vi "RTS Polarity CMD.vi"(7 "Station":u16=1 min=1 max=8 step=1, 8 "Error In":errorcluster, 11 "NewVal":T1) -> (0 "Error Out":errorcluster, 3 "Polarity CMD":string)   [LabVIEW 2016]
uses:
  Drivers/WAGO 750-881/Type Definitions/Wago Polarity Selector.ctl
  Drivers/WAGO 750-881/Type Definitions/Wago Input Commands.ctl
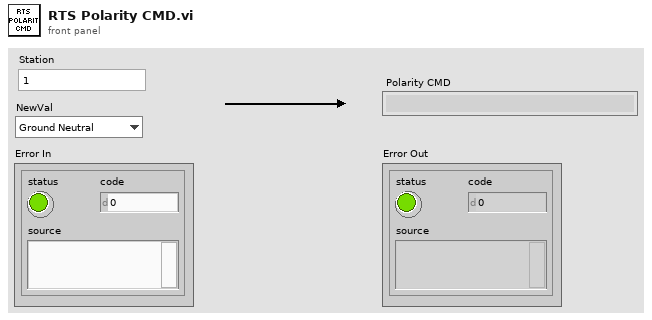
[diagram p1: front panel]
types:
  T1 = typedef "Wago Polarity Selector.ctl" = enum16{"Ground Neutral", "Ground Line"}
  T2 = typedef "Wago Input Commands.ctl" = u16
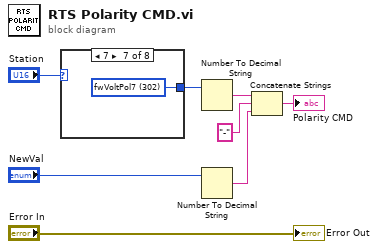
[diagram p0: block diagram]
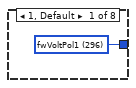
[diagram p2: hidden frame]
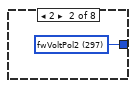
[diagram p3: hidden frame]
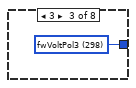
[diagram p4: hidden frame]
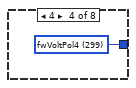
[diagram p5: hidden frame]
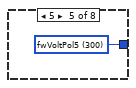
[diagram p6: hidden frame]
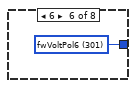
[diagram p7: hidden frame]
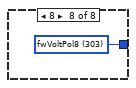
[diagram p8: hidden frame]
diagram:
  n1 = case shown="7" "Station" {
    tunnel: [w9 w10 w11 w12 w13 w14 w15 w16] -> w6
    frame 1, Default {
      w9 = T2 296 items=["fwS1Volt1"=0, "fwS1Volt2"=1, "fwS2Volt1"=2, "fwS2Volt2"=3, "fwS3Volt1"=4, "fwS3Volt2"=5, "fwS4Volt1"=6, "fwS4Volt2"=7, "fwS5Volt1"=8, "fwS5Volt2"=9, "fwS6Volt1"=10, "fwS6Volt2 "=11, "fwS7Volt1"=12, "fwS7Volt2"=13, "fwS8Volt1"=14, "fwS8Volt2"=15, "fwRoomHum"=16, "fwRoomTemp"=17, "fwAISpare1"=18, "fwAISpare2"=19, "fwSuppTemp"=20, "fwCoolTemp"=21, "fwDehumTemp"=22, "fwUnused"=23, "Bool Inputs"=24, "gwVoltRate1"=256, "gwVoltRate2"=257, "gwVoltRate3"=258, "gwVoltRate4"=259, "gwVoltRate5"=260, "gwVoltRate6"=261, "gwVoltRate7"=262, "gwVoltRate8"=263, "gwVoltWindow5/1"=264, "gwVoltWindow6/2"=265, "gwVoltWindow7/3"=266, "gwVoltWindow8/4"=267, "fwVoltSet1"=272, "fwVoltSet2"=273, "fwVoltSet3"=274, "fwVoltSet4"=275, "fwVoltSet5"=276, "fwVoltSet6"=277, "fwVoltSet7"=278, "fwVoltSet8"=279, "fwVoltRng1"=280, "fwVoltRng2"=281, "fwVoltRng3"=282, "fwVoltRng4"=283, "fwVoltRng5"=284, "fwVoltRng6"=285, "fwVoltRng7"=286, "fwVoltRng8"=287, "fwVoltPol1"=296, "fwVoltPol2"=297, "fwVoltPol3"=298, "fwVoltPol4"=299, "fwVoltPol5"=300, "fwVoltPol6"=301, "fwVoltPol7"=302, "fwVoltPol8"=303, "Rm1St1Dr1Cmd"=304, "Rm1St2Dr1Cmd"=305, "Rm1St3Dr1Cmd"=306, "Rm1St4Dr1Cmd"=307, "Rm1St5Dr1Cmd"=308, "Rm1St6Dr1Cmd"=309, "Rm1St7Dr1Cmd"=310, "Rm1St8Dr1Cmd"=311, "Rm1St1Dr2Cmd"=312, "Rm1St2Dr2Cmd"=313, "Rm1St3Dr2Cmd"=314, "Rm1St4Dr2Cmd"=315, "Rm1St5Dr2Cmd"=316, "Rm1St6Dr2Cmd"=317, "Rm1St7Dr2Cmd"=318, "Rm1St8Dr2Cmd"=319, "Rm1St1Dr3Cmd"=320, "Rm1St2Dr3Cmd"=321, "Rm1St3Dr3Cmd"=322, "Rm1St4Dr3Cmd"=323, "Rm1St5Dr3Cmd"=324, "Rm1St6Dr3Cmd"=325, "Rm1St7Dr3Cmd"=326, "Rm1St8Dr3Cmd"=327, "fwRmTempSP"=328, "fwRmHumSP"=329, "fwCoolTempSP"=330, "fwDehumTempSP"=331, "fwRmRun"=332, "fwRmOk"=333, "fwTesting"=334, "fwRmDryP"=335, "fwRmDryI"=336, "fwRmHumP"=337, "fwRmHumI"=338, "fwRmHeatP"=339, "fwRmHeatI"=340, "fwCoolTempP"=341, "fwCoolTempI"=342, "fwDehumTempP"=343, "fwDehumTempI"=344, "fwGndLeak1"=345, "fwGndLeak2"=346, "fwGndLeak3"=347, "fwGndLeak4"=348, "fwGndLeak5"=349, "fwGndLeak6"=350, "fwGndLeak7"=351, "fwGndLeak8"=352, "Rm1OpenerCmd"=353] ("Ring")
    }
    frame 2 {
      w10 = T2 297 items=["fwS1Volt1"=0, "fwS1Volt2"=1, "fwS2Volt1"=2, "fwS2Volt2"=3, "fwS3Volt1"=4, "fwS3Volt2"=5, "fwS4Volt1"=6, "fwS4Volt2"=7, "fwS5Volt1"=8, "fwS5Volt2"=9, "fwS6Volt1"=10, "fwS6Volt2 "=11, "fwS7Volt1"=12, "fwS7Volt2"=13, "fwS8Volt1"=14, "fwS8Volt2"=15, "fwRoomHum"=16, "fwRoomTemp"=17, "fwAISpare1"=18, "fwAISpare2"=19, "fwSuppTemp"=20, "fwCoolTemp"=21, "fwDehumTemp"=22, "fwUnused"=23, "Bool Inputs"=24, "gwVoltRate1"=256, "gwVoltRate2"=257, "gwVoltRate3"=258, "gwVoltRate4"=259, "gwVoltRate5"=260, "gwVoltRate6"=261, "gwVoltRate7"=262, "gwVoltRate8"=263, "gwVoltWindow5/1"=264, "gwVoltWindow6/2"=265, "gwVoltWindow7/3"=266, "gwVoltWindow8/4"=267, "fwVoltSet1"=272, "fwVoltSet2"=273, "fwVoltSet3"=274, "fwVoltSet4"=275, "fwVoltSet5"=276, "fwVoltSet6"=277, "fwVoltSet7"=278, "fwVoltSet8"=279, "fwVoltRng1"=280, "fwVoltRng2"=281, "fwVoltRng3"=282, "fwVoltRng4"=283, "fwVoltRng5"=284, "fwVoltRng6"=285, "fwVoltRng7"=286, "fwVoltRng8"=287, "fwVoltPol1"=296, "fwVoltPol2"=297, "fwVoltPol3"=298, "fwVoltPol4"=299, "fwVoltPol5"=300, "fwVoltPol6"=301, "fwVoltPol7"=302, "fwVoltPol8"=303, "Rm1St1Dr1Cmd"=304, "Rm1St2Dr1Cmd"=305, "Rm1St3Dr1Cmd"=306, "Rm1St4Dr1Cmd"=307, "Rm1St5Dr1Cmd"=308, "Rm1St6Dr1Cmd"=309, "Rm1St7Dr1Cmd"=310, "Rm1St8Dr1Cmd"=311, "Rm1St1Dr2Cmd"=312, "Rm1St2Dr2Cmd"=313, "Rm1St3Dr2Cmd"=314, "Rm1St4Dr2Cmd"=315, "Rm1St5Dr2Cmd"=316, "Rm1St6Dr2Cmd"=317, "Rm1St7Dr2Cmd"=318, "Rm1St8Dr2Cmd"=319, "Rm1St1Dr3Cmd"=320, "Rm1St2Dr3Cmd"=321, "Rm1St3Dr3Cmd"=322, "Rm1St4Dr3Cmd"=323, "Rm1St5Dr3Cmd"=324, "Rm1St6Dr3Cmd"=325, "Rm1St7Dr3Cmd"=326, "Rm1St8Dr3Cmd"=327, "fwRmTempSP"=328, "fwRmHumSP"=329, "fwCoolTempSP"=330, "fwDehumTempSP"=331, "fwRmRun"=332, "fwRmOk"=333, "fwTesting"=334, "fwRmDryP"=335, "fwRmDryI"=336, "fwRmHumP"=337, "fwRmHumI"=338, "fwRmHeatP"=339, "fwRmHeatI"=340, "fwCoolTempP"=341, "fwCoolTempI"=342, "fwDehumTempP"=343, "fwDehumTempI"=344, "fwGndLeak1"=345, "fwGndLeak2"=346, "fwGndLeak3"=347, "fwGndLeak4"=348, "fwGndLeak5"=349, "fwGndLeak6"=350, "fwGndLeak7"=351, "fwGndLeak8"=352, "Rm1OpenerCmd"=353] ("Ring")
    }
    frame 3 {
      w11 = T2 298 items=["fwS1Volt1"=0, "fwS1Volt2"=1, "fwS2Volt1"=2, "fwS2Volt2"=3, "fwS3Volt1"=4, "fwS3Volt2"=5, "fwS4Volt1"=6, "fwS4Volt2"=7, "fwS5Volt1"=8, "fwS5Volt2"=9, "fwS6Volt1"=10, "fwS6Volt2 "=11, "fwS7Volt1"=12, "fwS7Volt2"=13, "fwS8Volt1"=14, "fwS8Volt2"=15, "fwRoomHum"=16, "fwRoomTemp"=17, "fwAISpare1"=18, "fwAISpare2"=19, "fwSuppTemp"=20, "fwCoolTemp"=21, "fwDehumTemp"=22, "fwUnused"=23, "Bool Inputs"=24, "gwVoltRate1"=256, "gwVoltRate2"=257, "gwVoltRate3"=258, "gwVoltRate4"=259, "gwVoltRate5"=260, "gwVoltRate6"=261, "gwVoltRate7"=262, "gwVoltRate8"=263, "gwVoltWindow5/1"=264, "gwVoltWindow6/2"=265, "gwVoltWindow7/3"=266, "gwVoltWindow8/4"=267, "fwVoltSet1"=272, "fwVoltSet2"=273, "fwVoltSet3"=274, "fwVoltSet4"=275, "fwVoltSet5"=276, "fwVoltSet6"=277, "fwVoltSet7"=278, "fwVoltSet8"=279, "fwVoltRng1"=280, "fwVoltRng2"=281, "fwVoltRng3"=282, "fwVoltRng4"=283, "fwVoltRng5"=284, "fwVoltRng6"=285, "fwVoltRng7"=286, "fwVoltRng8"=287, "fwVoltPol1"=296, "fwVoltPol2"=297, "fwVoltPol3"=298, "fwVoltPol4"=299, "fwVoltPol5"=300, "fwVoltPol6"=301, "fwVoltPol7"=302, "fwVoltPol8"=303, "Rm1St1Dr1Cmd"=304, "Rm1St2Dr1Cmd"=305, "Rm1St3Dr1Cmd"=306, "Rm1St4Dr1Cmd"=307, "Rm1St5Dr1Cmd"=308, "Rm1St6Dr1Cmd"=309, "Rm1St7Dr1Cmd"=310, "Rm1St8Dr1Cmd"=311, "Rm1St1Dr2Cmd"=312, "Rm1St2Dr2Cmd"=313, "Rm1St3Dr2Cmd"=314, "Rm1St4Dr2Cmd"=315, "Rm1St5Dr2Cmd"=316, "Rm1St6Dr2Cmd"=317, "Rm1St7Dr2Cmd"=318, "Rm1St8Dr2Cmd"=319, "Rm1St1Dr3Cmd"=320, "Rm1St2Dr3Cmd"=321, "Rm1St3Dr3Cmd"=322, "Rm1St4Dr3Cmd"=323, "Rm1St5Dr3Cmd"=324, "Rm1St6Dr3Cmd"=325, "Rm1St7Dr3Cmd"=326, "Rm1St8Dr3Cmd"=327, "fwRmTempSP"=328, "fwRmHumSP"=329, "fwCoolTempSP"=330, "fwDehumTempSP"=331, "fwRmRun"=332, "fwRmOk"=333, "fwTesting"=334, "fwRmDryP"=335, "fwRmDryI"=336, "fwRmHumP"=337, "fwRmHumI"=338, "fwRmHeatP"=339, "fwRmHeatI"=340, "fwCoolTempP"=341, "fwCoolTempI"=342, "fwDehumTempP"=343, "fwDehumTempI"=344, "fwGndLeak1"=345, "fwGndLeak2"=346, "fwGndLeak3"=347, "fwGndLeak4"=348, "fwGndLeak5"=349, "fwGndLeak6"=350, "fwGndLeak7"=351, "fwGndLeak8"=352, "Rm1OpenerCmd"=353] ("Ring")
    }
    frame 4 {
      w12 = T2 299 items=["fwS1Volt1"=0, "fwS1Volt2"=1, "fwS2Volt1"=2, "fwS2Volt2"=3, "fwS3Volt1"=4, "fwS3Volt2"=5, "fwS4Volt1"=6, "fwS4Volt2"=7, "fwS5Volt1"=8, "fwS5Volt2"=9, "fwS6Volt1"=10, "fwS6Volt2 "=11, "fwS7Volt1"=12, "fwS7Volt2"=13, "fwS8Volt1"=14, "fwS8Volt2"=15, "fwRoomHum"=16, "fwRoomTemp"=17, "fwAISpare1"=18, "fwAISpare2"=19, "fwSuppTemp"=20, "fwCoolTemp"=21, "fwDehumTemp"=22, "fwUnused"=23, "Bool Inputs"=24, "gwVoltRate1"=256, "gwVoltRate2"=257, "gwVoltRate3"=258, "gwVoltRate4"=259, "gwVoltRate5"=260, "gwVoltRate6"=261, "gwVoltRate7"=262, "gwVoltRate8"=263, "gwVoltWindow5/1"=264, "gwVoltWindow6/2"=265, "gwVoltWindow7/3"=266, "gwVoltWindow8/4"=267, "fwVoltSet1"=272, "fwVoltSet2"=273, "fwVoltSet3"=274, "fwVoltSet4"=275, "fwVoltSet5"=276, "fwVoltSet6"=277, "fwVoltSet7"=278, "fwVoltSet8"=279, "fwVoltRng1"=280, "fwVoltRng2"=281, "fwVoltRng3"=282, "fwVoltRng4"=283, "fwVoltRng5"=284, "fwVoltRng6"=285, "fwVoltRng7"=286, "fwVoltRng8"=287, "fwVoltPol1"=296, "fwVoltPol2"=297, "fwVoltPol3"=298, "fwVoltPol4"=299, "fwVoltPol5"=300, "fwVoltPol6"=301, "fwVoltPol7"=302, "fwVoltPol8"=303, "Rm1St1Dr1Cmd"=304, "Rm1St2Dr1Cmd"=305, "Rm1St3Dr1Cmd"=306, "Rm1St4Dr1Cmd"=307, "Rm1St5Dr1Cmd"=308, "Rm1St6Dr1Cmd"=309, "Rm1St7Dr1Cmd"=310, "Rm1St8Dr1Cmd"=311, "Rm1St1Dr2Cmd"=312, "Rm1St2Dr2Cmd"=313, "Rm1St3Dr2Cmd"=314, "Rm1St4Dr2Cmd"=315, "Rm1St5Dr2Cmd"=316, "Rm1St6Dr2Cmd"=317, "Rm1St7Dr2Cmd"=318, "Rm1St8Dr2Cmd"=319, "Rm1St1Dr3Cmd"=320, "Rm1St2Dr3Cmd"=321, "Rm1St3Dr3Cmd"=322, "Rm1St4Dr3Cmd"=323, "Rm1St5Dr3Cmd"=324, "Rm1St6Dr3Cmd"=325, "Rm1St7Dr3Cmd"=326, "Rm1St8Dr3Cmd"=327, "fwRmTempSP"=328, "fwRmHumSP"=329, "fwCoolTempSP"=330, "fwDehumTempSP"=331, "fwRmRun"=332, "fwRmOk"=333, "fwTesting"=334, "fwRmDryP"=335, "fwRmDryI"=336, "fwRmHumP"=337, "fwRmHumI"=338, "fwRmHeatP"=339, "fwRmHeatI"=340, "fwCoolTempP"=341, "fwCoolTempI"=342, "fwDehumTempP"=343, "fwDehumTempI"=344, "fwGndLeak1"=345, "fwGndLeak2"=346, "fwGndLeak3"=347, "fwGndLeak4"=348, "fwGndLeak5"=349, "fwGndLeak6"=350, "fwGndLeak7"=351, "fwGndLeak8"=352, "Rm1OpenerCmd"=353] ("Ring")
    }
    frame 5 {
      w13 = T2 300 items=["fwS1Volt1"=0, "fwS1Volt2"=1, "fwS2Volt1"=2, "fwS2Volt2"=3, "fwS3Volt1"=4, "fwS3Volt2"=5, "fwS4Volt1"=6, "fwS4Volt2"=7, "fwS5Volt1"=8, "fwS5Volt2"=9, "fwS6Volt1"=10, "fwS6Volt2 "=11, "fwS7Volt1"=12, "fwS7Volt2"=13, "fwS8Volt1"=14, "fwS8Volt2"=15, "fwRoomHum"=16, "fwRoomTemp"=17, "fwAISpare1"=18, "fwAISpare2"=19, "fwSuppTemp"=20, "fwCoolTemp"=21, "fwDehumTemp"=22, "fwUnused"=23, "Bool Inputs"=24, "gwVoltRate1"=256, "gwVoltRate2"=257, "gwVoltRate3"=258, "gwVoltRate4"=259, "gwVoltRate5"=260, "gwVoltRate6"=261, "gwVoltRate7"=262, "gwVoltRate8"=263, "gwVoltWindow5/1"=264, "gwVoltWindow6/2"=265, "gwVoltWindow7/3"=266, "gwVoltWindow8/4"=267, "fwVoltSet1"=272, "fwVoltSet2"=273, "fwVoltSet3"=274, "fwVoltSet4"=275, "fwVoltSet5"=276, "fwVoltSet6"=277, "fwVoltSet7"=278, "fwVoltSet8"=279, "fwVoltRng1"=280, "fwVoltRng2"=281, "fwVoltRng3"=282, "fwVoltRng4"=283, "fwVoltRng5"=284, "fwVoltRng6"=285, "fwVoltRng7"=286, "fwVoltRng8"=287, "fwVoltPol1"=296, "fwVoltPol2"=297, "fwVoltPol3"=298, "fwVoltPol4"=299, "fwVoltPol5"=300, "fwVoltPol6"=301, "fwVoltPol7"=302, "fwVoltPol8"=303, "Rm1St1Dr1Cmd"=304, "Rm1St2Dr1Cmd"=305, "Rm1St3Dr1Cmd"=306, "Rm1St4Dr1Cmd"=307, "Rm1St5Dr1Cmd"=308, "Rm1St6Dr1Cmd"=309, "Rm1St7Dr1Cmd"=310, "Rm1St8Dr1Cmd"=311, "Rm1St1Dr2Cmd"=312, "Rm1St2Dr2Cmd"=313, "Rm1St3Dr2Cmd"=314, "Rm1St4Dr2Cmd"=315, "Rm1St5Dr2Cmd"=316, "Rm1St6Dr2Cmd"=317, "Rm1St7Dr2Cmd"=318, "Rm1St8Dr2Cmd"=319, "Rm1St1Dr3Cmd"=320, "Rm1St2Dr3Cmd"=321, "Rm1St3Dr3Cmd"=322, "Rm1St4Dr3Cmd"=323, "Rm1St5Dr3Cmd"=324, "Rm1St6Dr3Cmd"=325, "Rm1St7Dr3Cmd"=326, "Rm1St8Dr3Cmd"=327, "fwRmTempSP"=328, "fwRmHumSP"=329, "fwCoolTempSP"=330, "fwDehumTempSP"=331, "fwRmRun"=332, "fwRmOk"=333, "fwTesting"=334, "fwRmDryP"=335, "fwRmDryI"=336, "fwRmHumP"=337, "fwRmHumI"=338, "fwRmHeatP"=339, "fwRmHeatI"=340, "fwCoolTempP"=341, "fwCoolTempI"=342, "fwDehumTempP"=343, "fwDehumTempI"=344, "fwGndLeak1"=345, "fwGndLeak2"=346, "fwGndLeak3"=347, "fwGndLeak4"=348, "fwGndLeak5"=349, "fwGndLeak6"=350, "fwGndLeak7"=351, "fwGndLeak8"=352, "Rm1OpenerCmd"=353] ("Ring")
    }
    frame 6 {
      w14 = T2 301 items=["fwS1Volt1"=0, "fwS1Volt2"=1, "fwS2Volt1"=2, "fwS2Volt2"=3, "fwS3Volt1"=4, "fwS3Volt2"=5, "fwS4Volt1"=6, "fwS4Volt2"=7, "fwS5Volt1"=8, "fwS5Volt2"=9, "fwS6Volt1"=10, "fwS6Volt2 "=11, "fwS7Volt1"=12, "fwS7Volt2"=13, "fwS8Volt1"=14, "fwS8Volt2"=15, "fwRoomHum"=16, "fwRoomTemp"=17, "fwAISpare1"=18, "fwAISpare2"=19, "fwSuppTemp"=20, "fwCoolTemp"=21, "fwDehumTemp"=22, "fwUnused"=23, "Bool Inputs"=24, "gwVoltRate1"=256, "gwVoltRate2"=257, "gwVoltRate3"=258, "gwVoltRate4"=259, "gwVoltRate5"=260, "gwVoltRate6"=261, "gwVoltRate7"=262, "gwVoltRate8"=263, "gwVoltWindow5/1"=264, "gwVoltWindow6/2"=265, "gwVoltWindow7/3"=266, "gwVoltWindow8/4"=267, "fwVoltSet1"=272, "fwVoltSet2"=273, "fwVoltSet3"=274, "fwVoltSet4"=275, "fwVoltSet5"=276, "fwVoltSet6"=277, "fwVoltSet7"=278, "fwVoltSet8"=279, "fwVoltRng1"=280, "fwVoltRng2"=281, "fwVoltRng3"=282, "fwVoltRng4"=283, "fwVoltRng5"=284, "fwVoltRng6"=285, "fwVoltRng7"=286, "fwVoltRng8"=287, "fwVoltPol1"=296, "fwVoltPol2"=297, "fwVoltPol3"=298, "fwVoltPol4"=299, "fwVoltPol5"=300, "fwVoltPol6"=301, "fwVoltPol7"=302, "fwVoltPol8"=303, "Rm1St1Dr1Cmd"=304, "Rm1St2Dr1Cmd"=305, "Rm1St3Dr1Cmd"=306, "Rm1St4Dr1Cmd"=307, "Rm1St5Dr1Cmd"=308, "Rm1St6Dr1Cmd"=309, "Rm1St7Dr1Cmd"=310, "Rm1St8Dr1Cmd"=311, "Rm1St1Dr2Cmd"=312, "Rm1St2Dr2Cmd"=313, "Rm1St3Dr2Cmd"=314, "Rm1St4Dr2Cmd"=315, "Rm1St5Dr2Cmd"=316, "Rm1St6Dr2Cmd"=317, "Rm1St7Dr2Cmd"=318, "Rm1St8Dr2Cmd"=319, "Rm1St1Dr3Cmd"=320, "Rm1St2Dr3Cmd"=321, "Rm1St3Dr3Cmd"=322, "Rm1St4Dr3Cmd"=323, "Rm1St5Dr3Cmd"=324, "Rm1St6Dr3Cmd"=325, "Rm1St7Dr3Cmd"=326, "Rm1St8Dr3Cmd"=327, "fwRmTempSP"=328, "fwRmHumSP"=329, "fwCoolTempSP"=330, "fwDehumTempSP"=331, "fwRmRun"=332, "fwRmOk"=333, "fwTesting"=334, "fwRmDryP"=335, "fwRmDryI"=336, "fwRmHumP"=337, "fwRmHumI"=338, "fwRmHeatP"=339, "fwRmHeatI"=340, "fwCoolTempP"=341, "fwCoolTempI"=342, "fwDehumTempP"=343, "fwDehumTempI"=344, "fwGndLeak1"=345, "fwGndLeak2"=346, "fwGndLeak3"=347, "fwGndLeak4"=348, "fwGndLeak5"=349, "fwGndLeak6"=350, "fwGndLeak7"=351, "fwGndLeak8"=352, "Rm1OpenerCmd"=353] ("Ring")
    }
    frame 7 {
      w15 = T2 302 items=["fwS1Volt1"=0, "fwS1Volt2"=1, "fwS2Volt1"=2, "fwS2Volt2"=3, "fwS3Volt1"=4, "fwS3Volt2"=5, "fwS4Volt1"=6, "fwS4Volt2"=7, "fwS5Volt1"=8, "fwS5Volt2"=9, "fwS6Volt1"=10, "fwS6Volt2 "=11, "fwS7Volt1"=12, "fwS7Volt2"=13, "fwS8Volt1"=14, "fwS8Volt2"=15, "fwRoomHum"=16, "fwRoomTemp"=17, "fwAISpare1"=18, "fwAISpare2"=19, "fwSuppTemp"=20, "fwCoolTemp"=21, "fwDehumTemp"=22, "fwUnused"=23, "Bool Inputs"=24, "gwVoltRate1"=256, "gwVoltRate2"=257, "gwVoltRate3"=258, "gwVoltRate4"=259, "gwVoltRate5"=260, "gwVoltRate6"=261, "gwVoltRate7"=262, "gwVoltRate8"=263, "gwVoltWindow5/1"=264, "gwVoltWindow6/2"=265, "gwVoltWindow7/3"=266, "gwVoltWindow8/4"=267, "fwVoltSet1"=272, "fwVoltSet2"=273, "fwVoltSet3"=274, "fwVoltSet4"=275, "fwVoltSet5"=276, "fwVoltSet6"=277, "fwVoltSet7"=278, "fwVoltSet8"=279, "fwVoltRng1"=280, "fwVoltRng2"=281, "fwVoltRng3"=282, "fwVoltRng4"=283, "fwVoltRng5"=284, "fwVoltRng6"=285, "fwVoltRng7"=286, "fwVoltRng8"=287, "fwVoltPol1"=296, "fwVoltPol2"=297, "fwVoltPol3"=298, "fwVoltPol4"=299, "fwVoltPol5"=300, "fwVoltPol6"=301, "fwVoltPol7"=302, "fwVoltPol8"=303, "Rm1St1Dr1Cmd"=304, "Rm1St2Dr1Cmd"=305, "Rm1St3Dr1Cmd"=306, "Rm1St4Dr1Cmd"=307, "Rm1St5Dr1Cmd"=308, "Rm1St6Dr1Cmd"=309, "Rm1St7Dr1Cmd"=310, "Rm1St8Dr1Cmd"=311, "Rm1St1Dr2Cmd"=312, "Rm1St2Dr2Cmd"=313, "Rm1St3Dr2Cmd"=314, "Rm1St4Dr2Cmd"=315, "Rm1St5Dr2Cmd"=316, "Rm1St6Dr2Cmd"=317, "Rm1St7Dr2Cmd"=318, "Rm1St8Dr2Cmd"=319, "Rm1St1Dr3Cmd"=320, "Rm1St2Dr3Cmd"=321, "Rm1St3Dr3Cmd"=322, "Rm1St4Dr3Cmd"=323, "Rm1St5Dr3Cmd"=324, "Rm1St6Dr3Cmd"=325, "Rm1St7Dr3Cmd"=326, "Rm1St8Dr3Cmd"=327, "fwRmTempSP"=328, "fwRmHumSP"=329, "fwCoolTempSP"=330, "fwDehumTempSP"=331, "fwRmRun"=332, "fwRmOk"=333, "fwTesting"=334, "fwRmDryP"=335, "fwRmDryI"=336, "fwRmHumP"=337, "fwRmHumI"=338, "fwRmHeatP"=339, "fwRmHeatI"=340, "fwCoolTempP"=341, "fwCoolTempI"=342, "fwDehumTempP"=343, "fwDehumTempI"=344, "fwGndLeak1"=345, "fwGndLeak2"=346, "fwGndLeak3"=347, "fwGndLeak4"=348, "fwGndLeak5"=349, "fwGndLeak6"=350, "fwGndLeak7"=351, "fwGndLeak8"=352, "Rm1OpenerCmd"=353] ("Ring")
    }
    frame 8 {
      w16 = T2 303 items=["fwS1Volt1"=0, "fwS1Volt2"=1, "fwS2Volt1"=2, "fwS2Volt2"=3, "fwS3Volt1"=4, "fwS3Volt2"=5, "fwS4Volt1"=6, "fwS4Volt2"=7, "fwS5Volt1"=8, "fwS5Volt2"=9, "fwS6Volt1"=10, "fwS6Volt2 "=11, "fwS7Volt1"=12, "fwS7Volt2"=13, "fwS8Volt1"=14, "fwS8Volt2"=15, "fwRoomHum"=16, "fwRoomTemp"=17, "fwAISpare1"=18, "fwAISpare2"=19, "fwSuppTemp"=20, "fwCoolTemp"=21, "fwDehumTemp"=22, "fwUnused"=23, "Bool Inputs"=24, "gwVoltRate1"=256, "gwVoltRate2"=257, "gwVoltRate3"=258, "gwVoltRate4"=259, "gwVoltRate5"=260, "gwVoltRate6"=261, "gwVoltRate7"=262, "gwVoltRate8"=263, "gwVoltWindow5/1"=264, "gwVoltWindow6/2"=265, "gwVoltWindow7/3"=266, "gwVoltWindow8/4"=267, "fwVoltSet1"=272, "fwVoltSet2"=273, "fwVoltSet3"=274, "fwVoltSet4"=275, "fwVoltSet5"=276, "fwVoltSet6"=277, "fwVoltSet7"=278, "fwVoltSet8"=279, "fwVoltRng1"=280, "fwVoltRng2"=281, "fwVoltRng3"=282, "fwVoltRng4"=283, "fwVoltRng5"=284, "fwVoltRng6"=285, "fwVoltRng7"=286, "fwVoltRng8"=287, "fwVoltPol1"=296, "fwVoltPol2"=297, "fwVoltPol3"=298, "fwVoltPol4"=299, "fwVoltPol5"=300, "fwVoltPol6"=301, "fwVoltPol7"=302, "fwVoltPol8"=303, "Rm1St1Dr1Cmd"=304, "Rm1St2Dr1Cmd"=305, "Rm1St3Dr1Cmd"=306, "Rm1St4Dr1Cmd"=307, "Rm1St5Dr1Cmd"=308, "Rm1St6Dr1Cmd"=309, "Rm1St7Dr1Cmd"=310, "Rm1St8Dr1Cmd"=311, "Rm1St1Dr2Cmd"=312, "Rm1St2Dr2Cmd"=313, "Rm1St3Dr2Cmd"=314, "Rm1St4Dr2Cmd"=315, "Rm1St5Dr2Cmd"=316, "Rm1St6Dr2Cmd"=317, "Rm1St7Dr2Cmd"=318, "Rm1St8Dr2Cmd"=319, "Rm1St1Dr3Cmd"=320, "Rm1St2Dr3Cmd"=321, "Rm1St3Dr3Cmd"=322, "Rm1St4Dr3Cmd"=323, "Rm1St5Dr3Cmd"=324, "Rm1St6Dr3Cmd"=325, "Rm1St7Dr3Cmd"=326, "Rm1St8Dr3Cmd"=327, "fwRmTempSP"=328, "fwRmHumSP"=329, "fwCoolTempSP"=330, "fwDehumTempSP"=331, "fwRmRun"=332, "fwRmOk"=333, "fwTesting"=334, "fwRmDryP"=335, "fwRmDryI"=336, "fwRmHumP"=337, "fwRmHumI"=338, "fwRmHeatP"=339, "fwRmHeatI"=340, "fwCoolTempP"=341, "fwCoolTempI"=342, "fwDehumTempP"=343, "fwDehumTempI"=344, "fwGndLeak1"=345, "fwGndLeak2"=346, "fwGndLeak3"=347, "fwGndLeak4"=348, "fwGndLeak5"=349, "fwGndLeak6"=350, "fwGndLeak7"=351, "fwGndLeak8"=352, "Rm1OpenerCmd"=353] ("Ring")
    }
  }
  n2 = Number To Decimal String(number=w6) -> (decimal integer string=w3:string)  [unwired: 1 in]
  n3 = Number To Decimal String(number="NewVal") -> (decimal integer string=w1:string)  [unwired: 1 in]
  n4 = Concatenate Strings(w3, "-", w1) -> (→"Polarity CMD":string)
  "Error Out" <- "Error In"
